vi "arb_scale_sym.vi"(10 "wf":dbl[](array[numeric])) -> (2 "data":i16[](array[numeric]))   [LabVIEW 2017, in "wf.lvlib"]
uses:
  wf.lvlib
panel:
  out "Waveform Graph":i16[](graph)
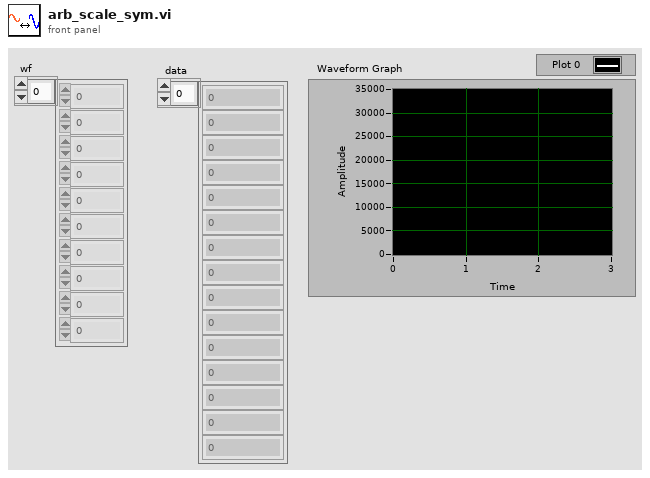
[diagram p1: front panel]
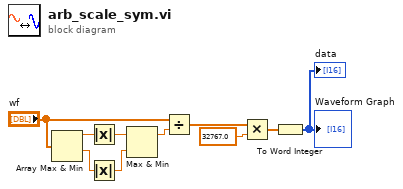
[diagram p0: block diagram]
diagram:
  n1 = Array Max & Min(array="wf") -> (max value=w6:dbl, min value=w7:dbl)  [unwired: 2 out]
  n2 = Absolute Value(x=w6) -> (abs(x)=w5:dbl)
  n3 = Absolute Value(x=w7) -> (abs(x)=w4:dbl)
  n4 = Max & Min(x=w5, y=w4) -> (max(x,y)=w3:dbl)  [unwired: 1 out]
  n5 = Divide(x="wf", y=w3) -> (x/y=w1:dbl[])
  n6 = Multiply(x=w1, y=32767.0) -> (x*y=w10:dbl[])
  n7 = To Word Integer(number=w10) -> (16bit integer=→"data" →"Waveform Graph":i16[])
